vi "getScriptEvent.vi"(8 "error in (no error)":errorcluster, 11 "ScanCreator in":refnum<class "ScanCreator.lvclass">) -> (0 "error out":errorcluster, 3 "ScanCreator out":refnum<class "ScanCreator.lvclass">)   [LabVIEW 2009, in "Views.lvlib" / "ScriptEditor.lvlib" / "ScanCreator.lvclass"]
uses:
  ScanCreator.lvclass
  ScanCreator.lvclass/ScanCreator.ctl
  Tools/Scripting/ScriptingEvent/ScriptEventList/ScriptEventList.lvclass
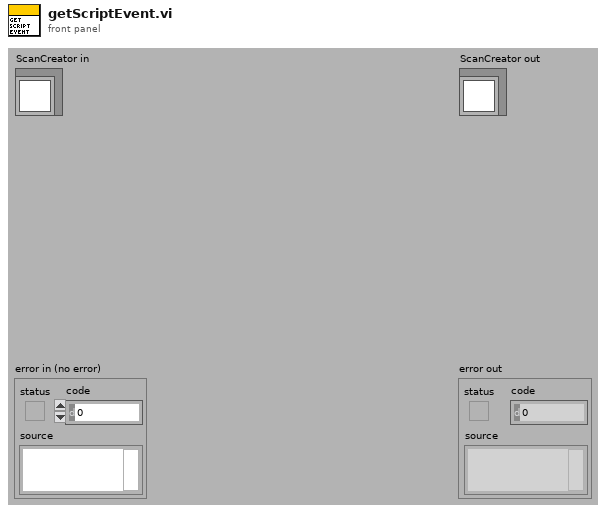
[diagram p1: front panel]
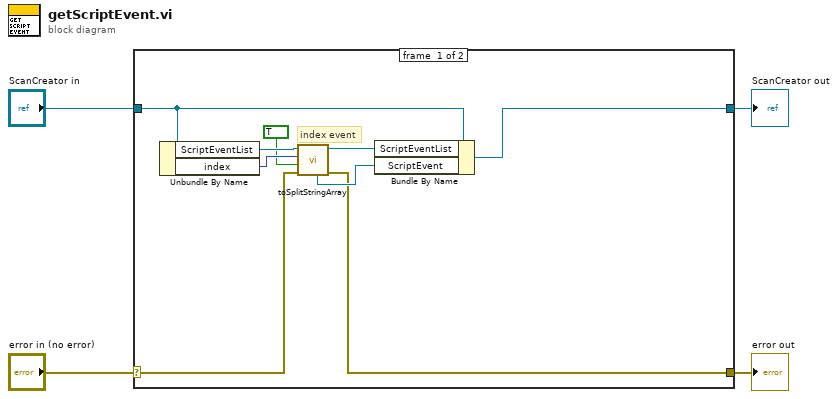
[diagram p0: block diagram]
diagram:
  n1 = case shown="No Error" "error in (no error)" {
    selector: "error in (no error)" -> [w11 w15]
    tunnel: [w5 w15] -> w3
    tunnel: [w7 w14] -> w1
    tunnel: "ScanCreator in" -> [w8 w14]
    frame #0 {
      # "index event"
      n2 = Unbundle By Name(w8) -> ("ScriptEventList"=w13:refnum<class "ScriptEventList.lvclass">, "index"=w12:i16)
      n3 = call "toSplitStringArray.vi"("error in (no error)"=w11, "editing?"=TRUE, "splitIndex"=w12, "ScriptEventList in"=w13) -> ("error out"=w5:errorcluster, "ScriptEventList out"=w9:refnum<class "ScriptEventList.lvclass">, "indexedScriptEvent"=w6:refnum<class "ScriptEvent.lvclass">)  [unwired: 3 in, 2 out]
      n4 = Bundle By Name(cluster=w8, "ScriptEventList"=w9, "ScriptEvent"=w6) -> (w7:refnum<class "ScanCreator.lvclass">)
    }
    frame #1 {
    }
  }
  "error out" <- w3
  "ScanCreator out" <- w1
